vi "RangeMeasureLimitInitialize.vi"(8 "error in":errorcluster, 10 "ComparisonType":T1, 11 "RangeMeasureLimit in":refnum<class "RangeMeasureLimit.lvclass">) -> (0 "error out":errorcluster, 3 "RangeMeasureLimit out":refnum<class "RangeMeasureLimit.lvclass">)   [LabVIEW 2021, in "ProligentXMLGenerator.lvlib" / "RangeMeasureLimit.lvclass"]
uses:
  RangeMeasureLimit.lvclass
  RangeMeasureLimit.lvclass/RangeMeasureLimit.ctl
  ComparisonType.ctl
  Data.ctl
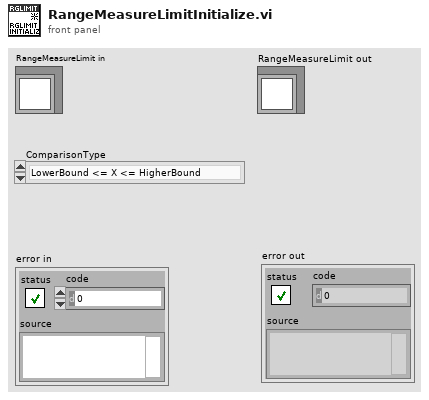
[diagram p1: front panel]
types:
  T1 = typedef "ProligentXMLGenerator.lvlib/RangeMeasureLimit.lvclass/ComparisonType.ctl" = enum16{"LowerBound <= X <= HigherBound", "LowerBound < X <= HigherBound", "LowerBound <= X < HigherBound", "LowerBound < X < HigherBound", "LowerBound <= X", "LowerBound < X", "X <= HigherBound", "X < HigherBound", "X == HigherBound", "X != HigherBound", "X <= LowerBound OR HigherBound <= X", "X < LowerBound OR HigherBound <= X", "X <= LowerBound OR HigherBound < X", "X < LowerBound OR HigherBound < X"}
  T2 = typedef "ProligentXMLGenerator.lvlib/RangeMeasureLimit.lvclass/Data.ctl" = cluster{"ComparisonType":T1}
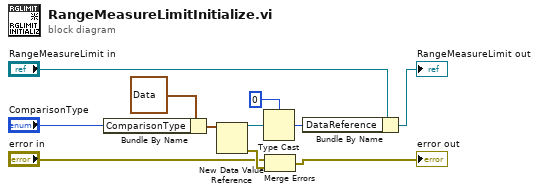
[diagram p0: block diagram]
diagram:
  n1 = Bundle By Name(cluster=T2 {"ComparisonType"=enum."LowerBound <= X <= HigherBound"} ("Data"), "ComparisonType"="ComparisonType") -> (w7:T2)
  n2 = New Data Value Reference(data value=w7) -> (data value reference=w8:refnum<data-value>, error out=w11:errorcluster)  [unwired: 1 in]
  n3 = Type Cast(type=u64 0, x=w8) -> (*(type *) &x=w10:u64)
  n4 = Merge Errors("error in", w11) -> (→"error out":errorcluster)
  n5 = Bundle By Name(cluster="RangeMeasureLimit in", "DataReference"=w10) -> (→"RangeMeasureLimit out":refnum<class "RangeMeasureLimit.lvclass">)
